vi "Data Replay Loop Page.vi"(8 "error in (no error)":errorcluster, 11 "Node Ptr":T1 format="%.0x") -> (0 "error out":errorcluster)   [LabVIEW 2011, in "Engine Sim System Explorer.lvlib"]
uses:
  Engine Sim System Explorer.lvlib
  <vilib>/NI Veristand/Custom Device API/Custom Device Item Ref.ctl
  Shared/Engine Simulation Global.vi
  <vilib>/NI Veristand/Custom Device API/Get Item Property (Double).vi
  <vilib>/rvi/Analysis/host/Private/Sample Rate To Loop Time (ticks).vi
  <vilib>/NI Veristand/Custom Device API/Set Item Property (Double).vi
  <vilib>/NI Veristand/Custom Device API/Custom Device API.lvlib
  Engine Simulation Shared.lvlib
  <vilib>/rvi/Analysis/host/Public/NI_FpgaMspHost.lvlib
panel:
  out "Actual Loop Rate (Hz)":dbl format="%#.10f"
  in  "Loop Rate (Hz)":dbl format="%#_10f"
  in  "SHDocVw.IWebBrowser2":refnum<k7>(container)
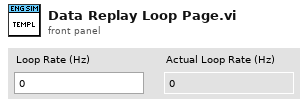
[diagram p1: front panel]
types:
  T1 = typedef "Custom Device API.lvlib/Custom Device Item Ref.ctl" = u64
  T2 = typedef "Custom Device API.lvlib/Custom Device Commands.ctl" = enum16{"Default", "Item renamed", "Shutdown", "Dynamic button pressed"}
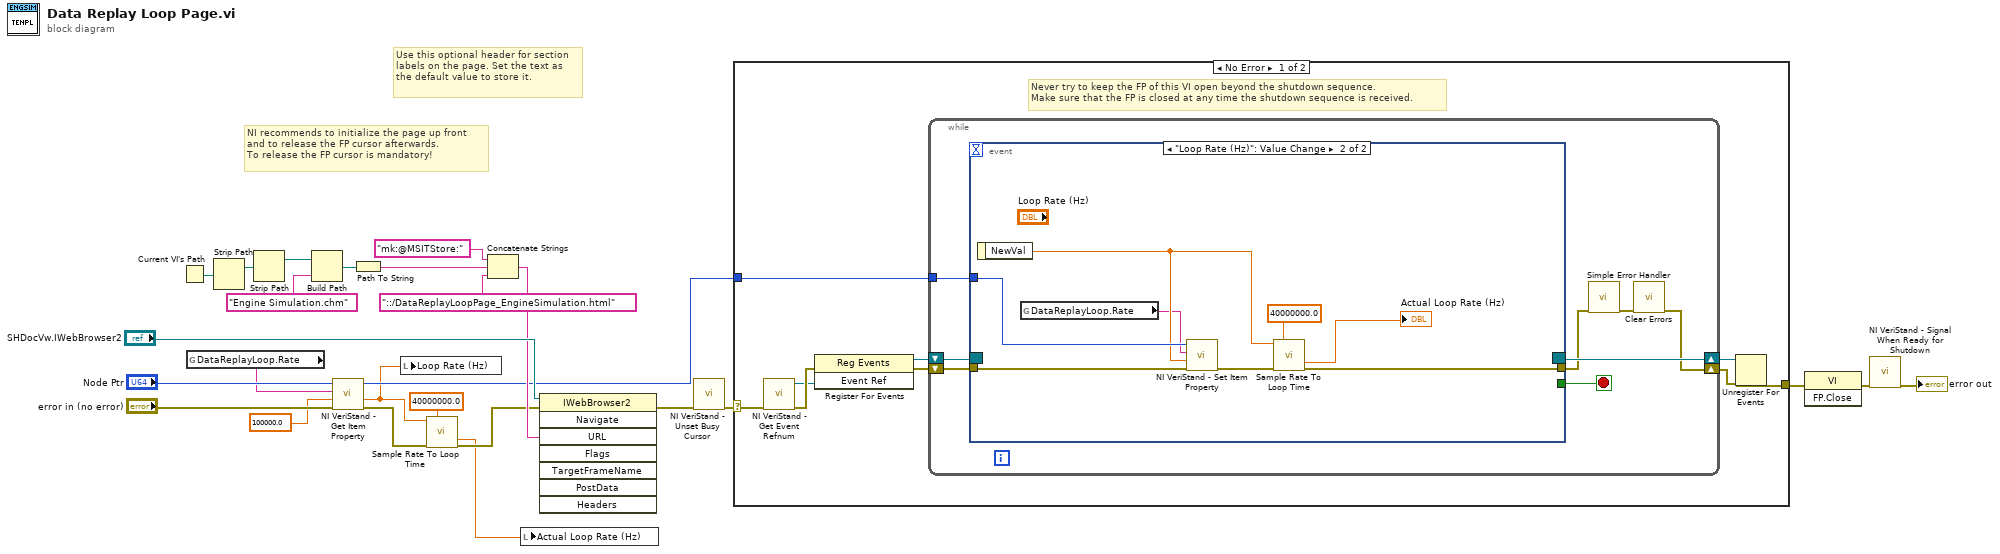
[diagram p0: block diagram]
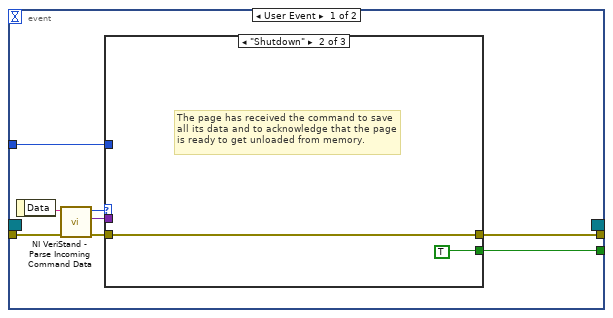
[diagram p2: hidden frame]
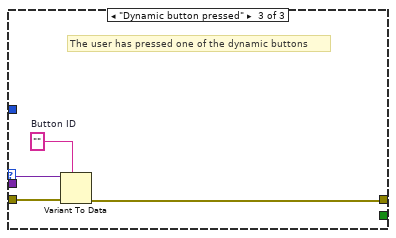
[diagram p4: hidden frame]
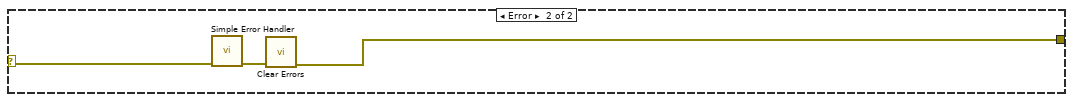
[diagram p5: hidden frame]
diagram:
  # "Use this optional header for section labels on the page. Set the text as the default value to store it."
  # "NI recommends to initialize the page up front\nand to release the FP cursor afterwards.\nTo release the FP cursor is mandatory!"
  n1 = Current VI's Path() -> (path=w12:path)
  n2 = global read "Engine Simulation Global.vi" "DataReplayLoop.Rate"() -> (w7:string)
  n3 = Strip Path(path=w12) -> (stripped path=w13:path)  [unwired: 1 out]
  n4 = Strip Path(path=w13) -> (stripped path=w18:path)  [unwired: 1 out]
  n5 = Build Path(base path=w18, name or relative path="Engine Simulation.chm") -> (appended path=w16:path)
  n6 = call-poly <vilib>:"NI VeriStand - Get Item Property.vi"("error in (no error)"="error in (no error)", "Default Value"=100000.0 ("Loop Rate (Hz)"), "Property Name"=w7, "Item Ref in"="Node Ptr") -> ("error out"=w5:errorcluster, "Value"=w3:dbl, "Item Ref out"=w8:T1)  [unwired: 4 in, 1 out]
  n7 = Path To String(path=w16) -> (string=w15:string)
  n8 = local write "Loop Rate (Hz)"(w3) -> ()
  n9 = call-poly <vilib>:"Sample Rate To Loop Time.vi"("sample rate (S/s)"=w3, "FPGA clock rate (Hz)"=40000000.0, "error in (no error)"=w5) -> ("actual sample rate (S/s)"=w1:dbl, "error out"=w2:errorcluster)  [unwired: 10 in, 1 out]
  n10 = Concatenate Strings("mk:@MSITStore:" ("string"), w15, "::/DataReplayLoopPage_EngineSimulation.html" ("name or relative path")) -> (w10:string)
  n11 = local write "Actual Loop Rate (Hz)"(w1) -> ()
  n12 = invoke class="IWebBrowser2" method="Navigate"(reference="SHDocVw.IWebBrowser2", error in=w2, "URL"=w10) -> (error out=w22:errorcluster)  [unwired: 5 in, 7 out]
  n13 = call <vilib>:"NI VeriStand - Unset Busy Cursor.vi"("error in (no error)"=w22) -> ("error out"=w21:errorcluster)  [unwired: 10 out]
  n14 = case shown="No Error" w21 {
    selector: w21 -> [w26 w68]
    tunnel: [w31 w66] -> w25
    tunnel: w8 -> [w27 _]
    frame No Error {
      # "Never try to keep the FP of this VI open beyond the shutdown sequence.\nMake sure that the FP is closed at any time the shutdown sequence is received."
      n15 = call <vilib>:"NI VeriStand - Get Event Refnum.vi"("error in (no error)"=w26) -> ("error out"=w34:errorcluster, "Event Ref"=w30:refnum<user-event>)  [unwired: 9 out]
      n16 = register-events(error in=w34, w30) -> (reference out=w28:refnum<event-registration>, error out=w29:errorcluster)  [unwired: 1 in]
      n17 = while {
        tunnel: w27 -> [w38]
        shift-right: [w35] -> w32
        shift-left: w29 -> [w41]
        shift-right: [w42] -> w33
        shift-left: w28 -> [w40]
        stop <- w39 stop-if-true
        n18 = event shown="[1] \"Loop Rate (Hz)\": Value Change" {
          selector: w40 -> [_ _]
          dyn-events: [_ _] -> w42
          timeout: _ -> [_ _]
          tunnel: w41 -> [w50 w65]
          tunnel: [w46 _] -> w39
          tunnel: [w45 w62] -> w37
          tunnel: w38 -> [w44 w60]
          event User Event {
            n19 = event-data() -> ("Data"=w49:string)  [unwired: 1 out]
            n20 = call <vilib>:"NI VeriStand - Parse Incoming Command Data.vi"("error in (no error)"=w50, "Incoming data"=w49) -> ("error out"=w48:errorcluster, "Outgoing data"=w43:variant, "Action"=w47:T2)  [unwired: 7 out]
            n21 = case shown="\"Shutdown\"" w47 {
              tunnel: w48 -> [w51 w52 w57]
              tunnel: [_ TRUE _] -> w46
              tunnel: [w51 w52 w54] -> w45
              tunnel: w44 -> [_ _ _]
              tunnel: w43 -> [_ _ w56]
              frame "Default", Default {
              }
              frame "Shutdown" {
                # "The page has received the command to save all its data and to acknowledge that the page is ready to get unloaded from memory."
              }
              frame "Dynamic button pressed" {
                w55 = ""  # Button ID
                # "The user has pressed one of the dynamic buttons"
                n22 = Variant To Data(error in=w57, type=w55, Variant=w56) -> (error out=w54:errorcluster)  [unwired: 1 out]
              }
            }
          }
          event "Loop Rate (Hz)": Value Change {
            n23 = event-data() -> ("NewVal"=w59:dbl)  [unwired: 1 out]
            n24 = global read "Engine Simulation Global.vi" "DataReplayLoop.Rate"() -> (w58:string)
            n25 = call-poly <vilib>:"NI VeriStand - Set Item Property.vi"("error in (no error)"=w65, "Value"=w59, "Property Name"=w58, "Item Ref in"=w60) -> ("error out"=w61:errorcluster)  [unwired: 5 in, 2 out]
            n26 = call-poly <vilib>:"Sample Rate To Loop Time.vi"("sample rate (S/s)"=w59, "FPGA clock rate (Hz)"=40000000.0, "error in (no error)"=w61) -> ("actual sample rate (S/s)"=→"Actual Loop Rate (Hz)":dbl, "error out"=w62:errorcluster)  [unwired: 10 in, 1 out]
          }
        }
        n27 = call <vilib>:"Simple Error Handler.vi"("error in (no error)"=w37) -> ("error out"=w36:errorcluster)  [unwired: 1 in, 7 out]
        n28 = call <vilib>:"Clear Errors.vi"("error in (no error)"=w36) -> ("error out"=w35:errorcluster)  [unwired: 6 out]
      }
      n29 = Unregister For Events(event registration refnum=w33, error in=w32) -> (error out=w31:errorcluster)
    }
    frame Error {
      n30 = call <vilib>:"Simple Error Handler.vi"("error in (no error)"=w68) -> ("error out"=w67:errorcluster)  [unwired: 1 in, 7 out]
      n31 = call <vilib>:"Clear Errors.vi"("error in (no error)"=w67) -> ("error out"=w66:errorcluster)  [unwired: 6 out]
    }
  }
  n32 = invoke class="VI" method="FP.Close"(error in=w25) -> (error out=w24:errorcluster)  [unwired: 2 in, 2 out]
  n33 = call <vilib>:"NI VeriStand - Signal When Ready for Shutdown.vi"("error in (no error)"=w24) -> ("error out"=→"error out":errorcluster)  [unwired: 10 out]
